vi "channel operation tests.vi"() -> ()   [LabVIEW 2013, in "scan engine tests.lvlib"]
uses:
  scan engine tests.lvlib
  configuration/Scan Engine configuration.lvclass
panel:
  out "no err":errorcluster
  out "channels match":bool
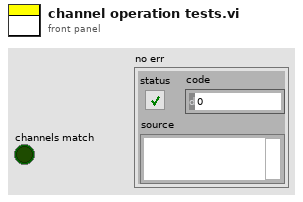
[diagram p1: front panel]
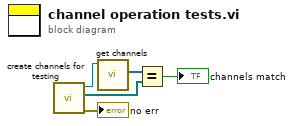
[diagram p0: block diagram]
diagram:
  n1 = call "create channels for testing.vi"() -> ("error out"=→"no err":errorcluster, "chans"=w3:refnum<class "TBM channel.lvclass">[], "Scan Engine configuration out"=w2:refnum<class "Scan Engine configuration.lvclass">)  [unwired: 7 in, 2 out]
  n2 = call-dynamic "get channels.vi"("module configuration in"=w2) -> ("channels"=w5:refnum<class "TBM channel.lvclass">[])  [unwired: 9 in, 1 out]
  n3 = Equal?(x=w5, y=w3) -> (x = y?=→"channels match":bool)
